vi "ReadTransducer.vi"(2 "error in (no error)":errorcluster, 3 "file path":path) -> (0 "error out":errorcluster, 1 "sensor":T1(array[cluster]))   [LabVIEW 2011]
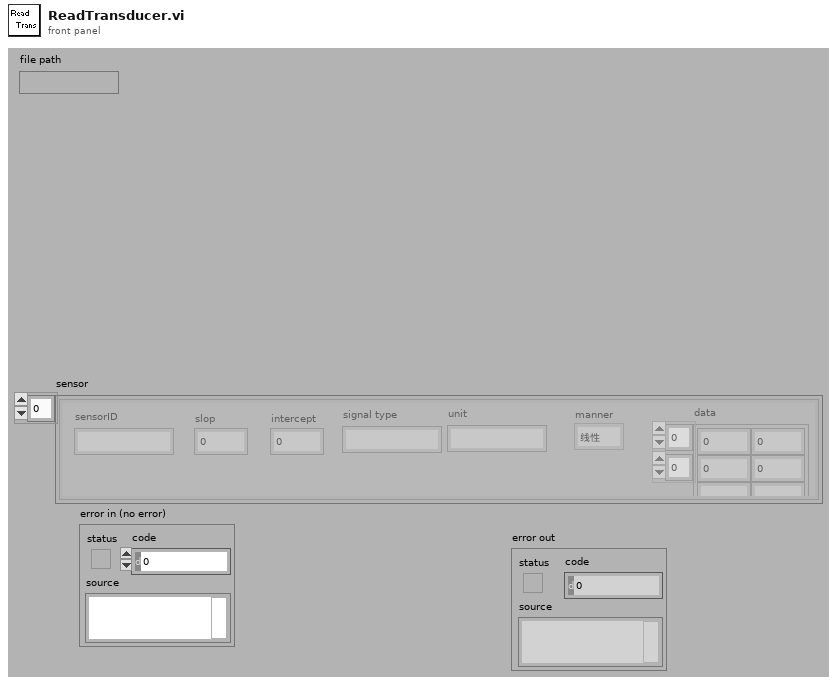
[diagram p1: front panel]
types:
  T1 = cluster{"manner":enum16{"线性", "查表"}, "data":dbl[][], "slop":dbl, "intercept":dbl, "sensorID":string, "signal type":string, "unit":string}[]
  T2 = cluster{"manner":enum16{"线性", "查表"}, "data":dbl[][], "slop":dbl, "intercept":dbl, "sensorID":string, "signal type":string, "unit":string}
  T3 = enum16{"big-endian, network order", "native, host order", "little-endian"}
  T4 = enum16{"open", "replace", "create", "open or create", "replace or create", "replace or create with confirmation"}
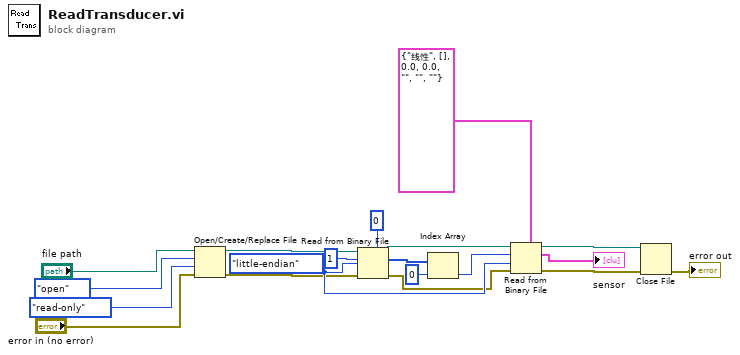
[diagram p0: block diagram]
diagram:
  w9 = T3."little-endian" ("byte order (0:big-endian, network order)")
  n1 = Open/Create/Replace File(file path (use dialog)="file path", error in="error in (no error)", operation (0:open)=T4."open", access (0:read/write)=enum16{"read/write", "read-only", "write-only"}."read-only") -> (refnum out=w16:refnum<file>, error out=w5:errorcluster)  [unwired: 3 out]
  n2 = Read from Binary File(5:0, 8:w5, 9:w9, 10:1 ("count"), 11:w16) -> (0:w4:errorcluster, 2:w13:i32[], 3:w11:refnum<file>)  [unwired: 2 out]
  n3 = Index Array(array=w13, index=0) -> (element=w10:i32)
  n4 = Read from Binary File(5:T2 {"manner"=enum."线性", "data"=[], "slop"=0.0, "intercept"=0.0, "sensorID"="", "signal type"="", "unit"=""} ("Sensor"), 8:w4, 9:w9, 10:w10, 11:w11) -> (0:w3:errorcluster, 2:→"sensor":T1, 3:w8:refnum<file>)  [unwired: 2 out]
  n5 = Close File(refnum=w8, error in=w3) -> (error out=→"error out":errorcluster)  [unwired: 1 out]
